vi "CalibrationFileIO.vi"(4 "Current Image Pixels":cluster{"X Pixels":i32, "Y Pixels":i32}, 6 "Calibration Type":string, 7 "CalibrationFileIO_command":enum16{"WriteSettings", "ReadSettings"}(ring), 8 "Pixel Mapping to Write":cluster{"X-PixelMap":i32[], "Y-PixelMap":i32[]}, 9 "Common Parameters IN":T1={"X.ZOOM.Compensation"=1.0, "Y.ZOOM.Compensation"=1.0, "Reso_Phase.Correction"=0.0}, 10 "Calibration paramaters_IN":T2, 11 "configuration file path":path) -> (1 "Common Parameters OUT":T1, 2 "Param Matches during a read":i32, 3 "Calibration paramaters_OUT":T2)   [LabVIEW 2012]
uses:
  Custom Controls and Typedefs/Calibration paramaters to Save.ctl
  Custom Controls and Typedefs/Calibration_commonParams.ctl
  Custom Controls and Typedefs/FGV_CalibrationKeyParams_Actions.ctl
  <vilib>/Utility/config.llb/Write Key (String).vi
  <vilib>/Utility/config.llb/Write Key (Boolean).vi
  <vilib>/Utility/config.llb/Write Key (Double).vi
  <vilib>/Utility/config.llb/Write Key (I32).vi
  <vilib>/Utility/config.llb/Read Key (Boolean).vi
  <vilib>/Utility/config.llb/Read Key (Double).vi
  <vilib>/Utility/config.llb/Read Key (I32).vi
  <vilib>/Utility/config.llb/Read Key (String).vi
  <vilib>/Utility/config.llb/NI_LVConfig.lvlib
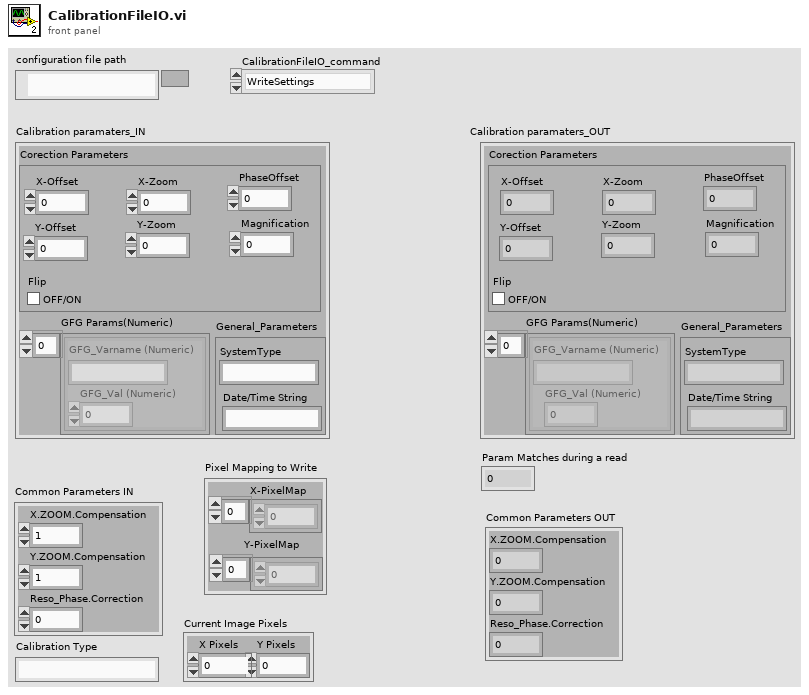
[diagram p1: front panel]
types:
  T1 = typedef "Calibration_commonParams.ctl" = cluster{"X.ZOOM.Compensation":dbl, "Y.ZOOM.Compensation":dbl, "Reso_Phase.Correction":dbl}
  T2 = typedef "Calibration paramaters to Save.ctl" = cluster{"General_Parameters":cluster{"SystemType":string, "Date/Time String":string}, "Corection Parameters":cluster{"X-Offset":i32, "Y-Offset":i32, "X-Zoom":dbl, "Y-Zoom":dbl, "PhaseOffset":dbl, "Magnification":dbl, "Flip":bool}, "GFG Params(Numeric)":cluster{"GFG_Varname (Numeric)":string, "GFG_Val (Numeric)":dbl}[]}
  T3 = typedef "FGV_CalibrationKeyParams_Actions.ctl" = enum16{"Initialize", "Grab From SciScan and Store", "Read Parameters", "ReadGFGValue"}
  T4 = typedef "NI_LVConfig.lvlib/Config Data RefNum.ctl" = refnum<k1>
  T5 = typedef "Calibration Key Param structure.ctl" = cluster{"GFG Variable Name":string, "Data Type":T6, "Value":variant}
  T6 = typedef "VariantType.lvlib/Type.ctl" = enum8{"Invalid Type", "Void", "I8", "I16", "I32", "I64", "U8", "U16", "U32", "U64", "Single Float", "Double Float", "Extended Float", "Single Complex", "Double Complex", "Extended Complex", "Enum U8", "Enum U16", "Enum U32", "Enum U64", "Single Float With Unit", "Double Float With Unit", "Extended Float With Unit", "Single Complex with Unit", "Double Complex with Unit", "Extended Complex with Unit", "Boolean", "String", "Path", "Picture", "Tag", "Array", "Cluster", "Variant", "LV Variant", "Waveform", "Timestamp", "Digital Waveform", "Digital Data", "ExpressData", "Refnum", "External Data", "VI", "Poly VI", "LabVIEW Class Instance", "Fixed Point"}
  T7 = cluster{"Key Parameters Array":T5[], "Key String":string}
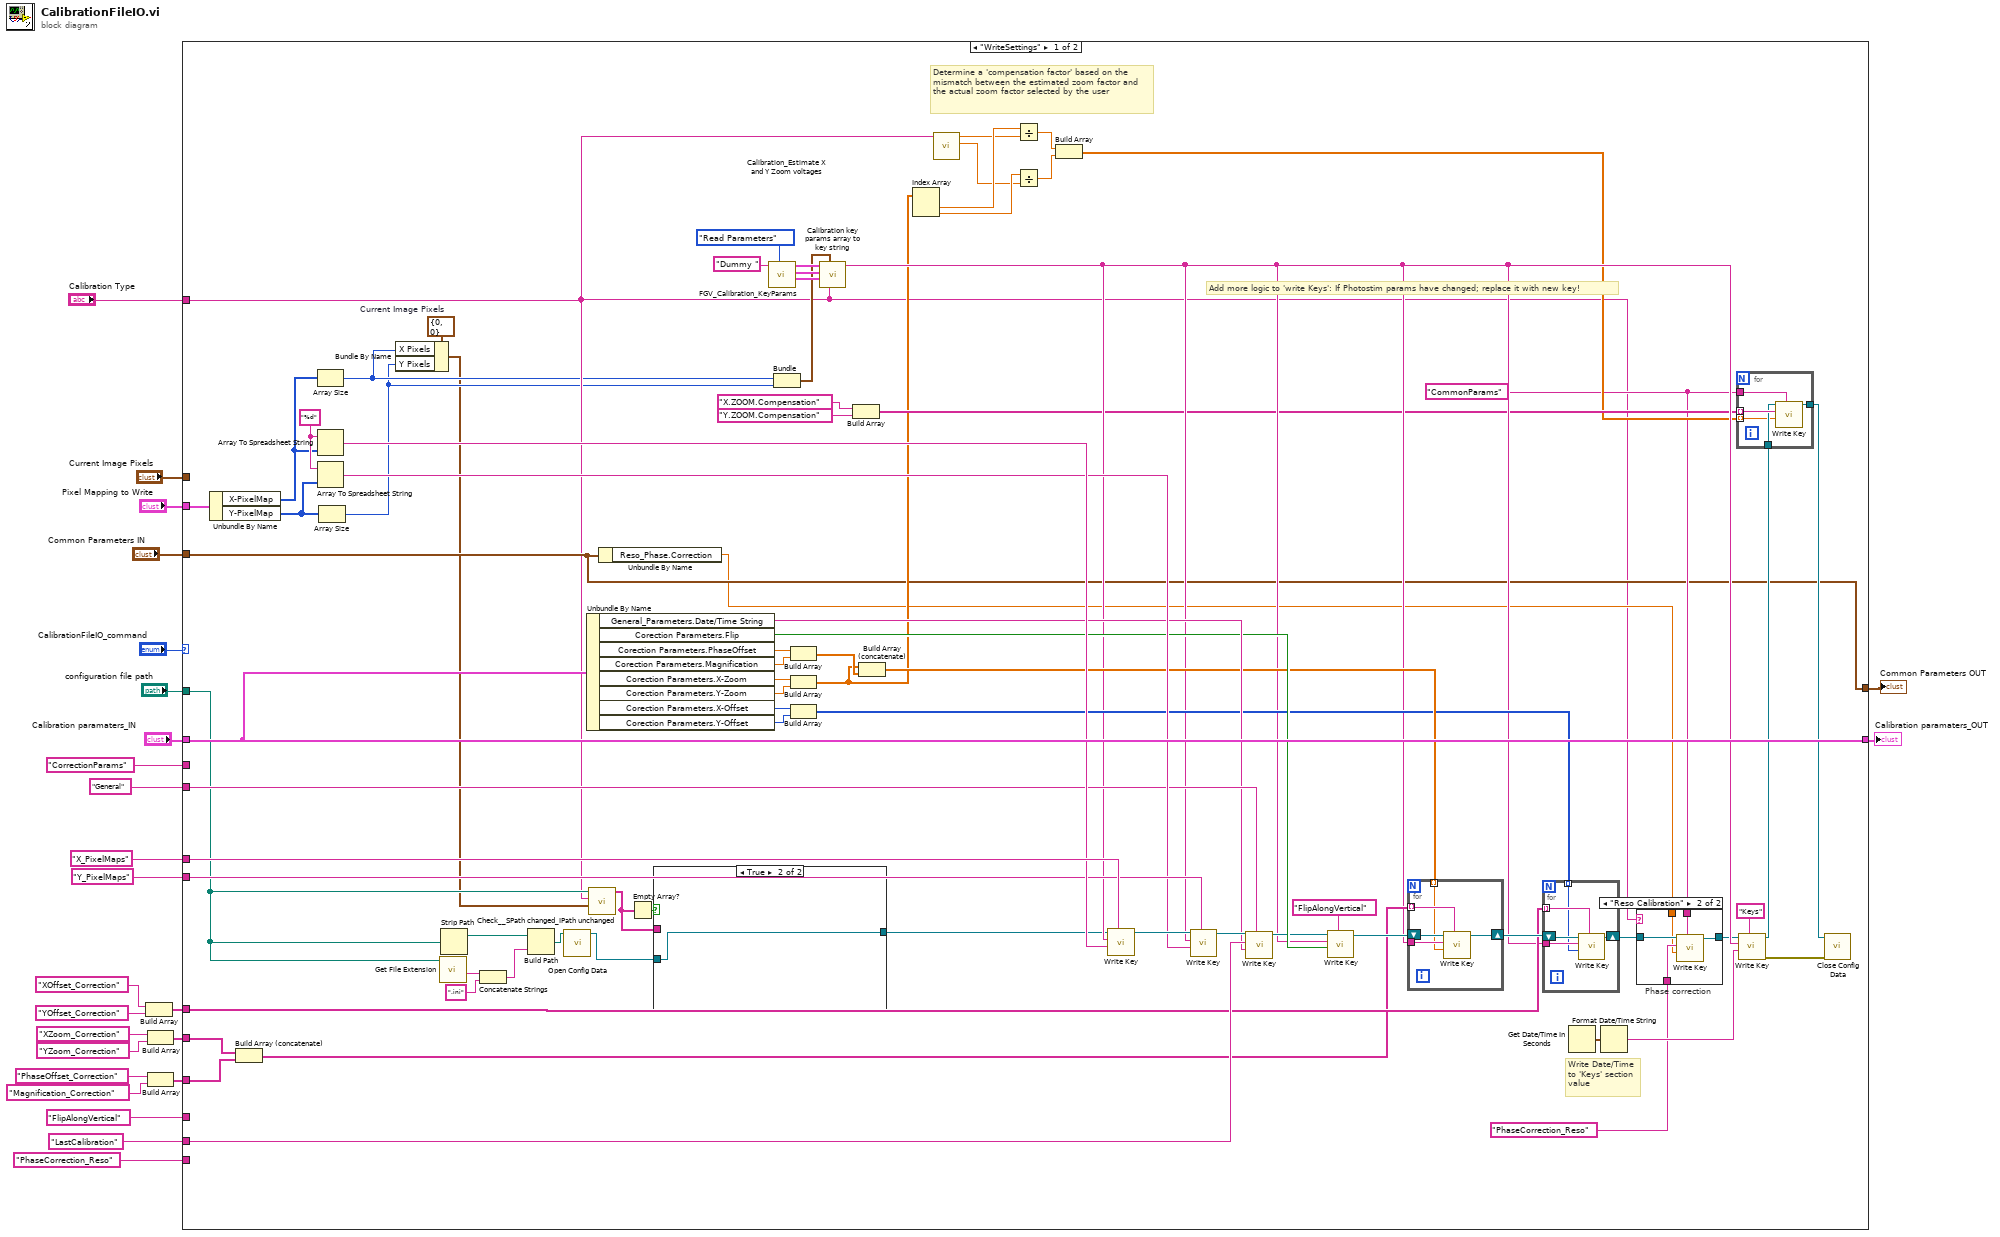
[diagram p0: block diagram]
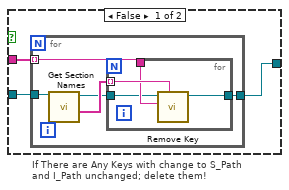
[diagram p2: hidden frame]
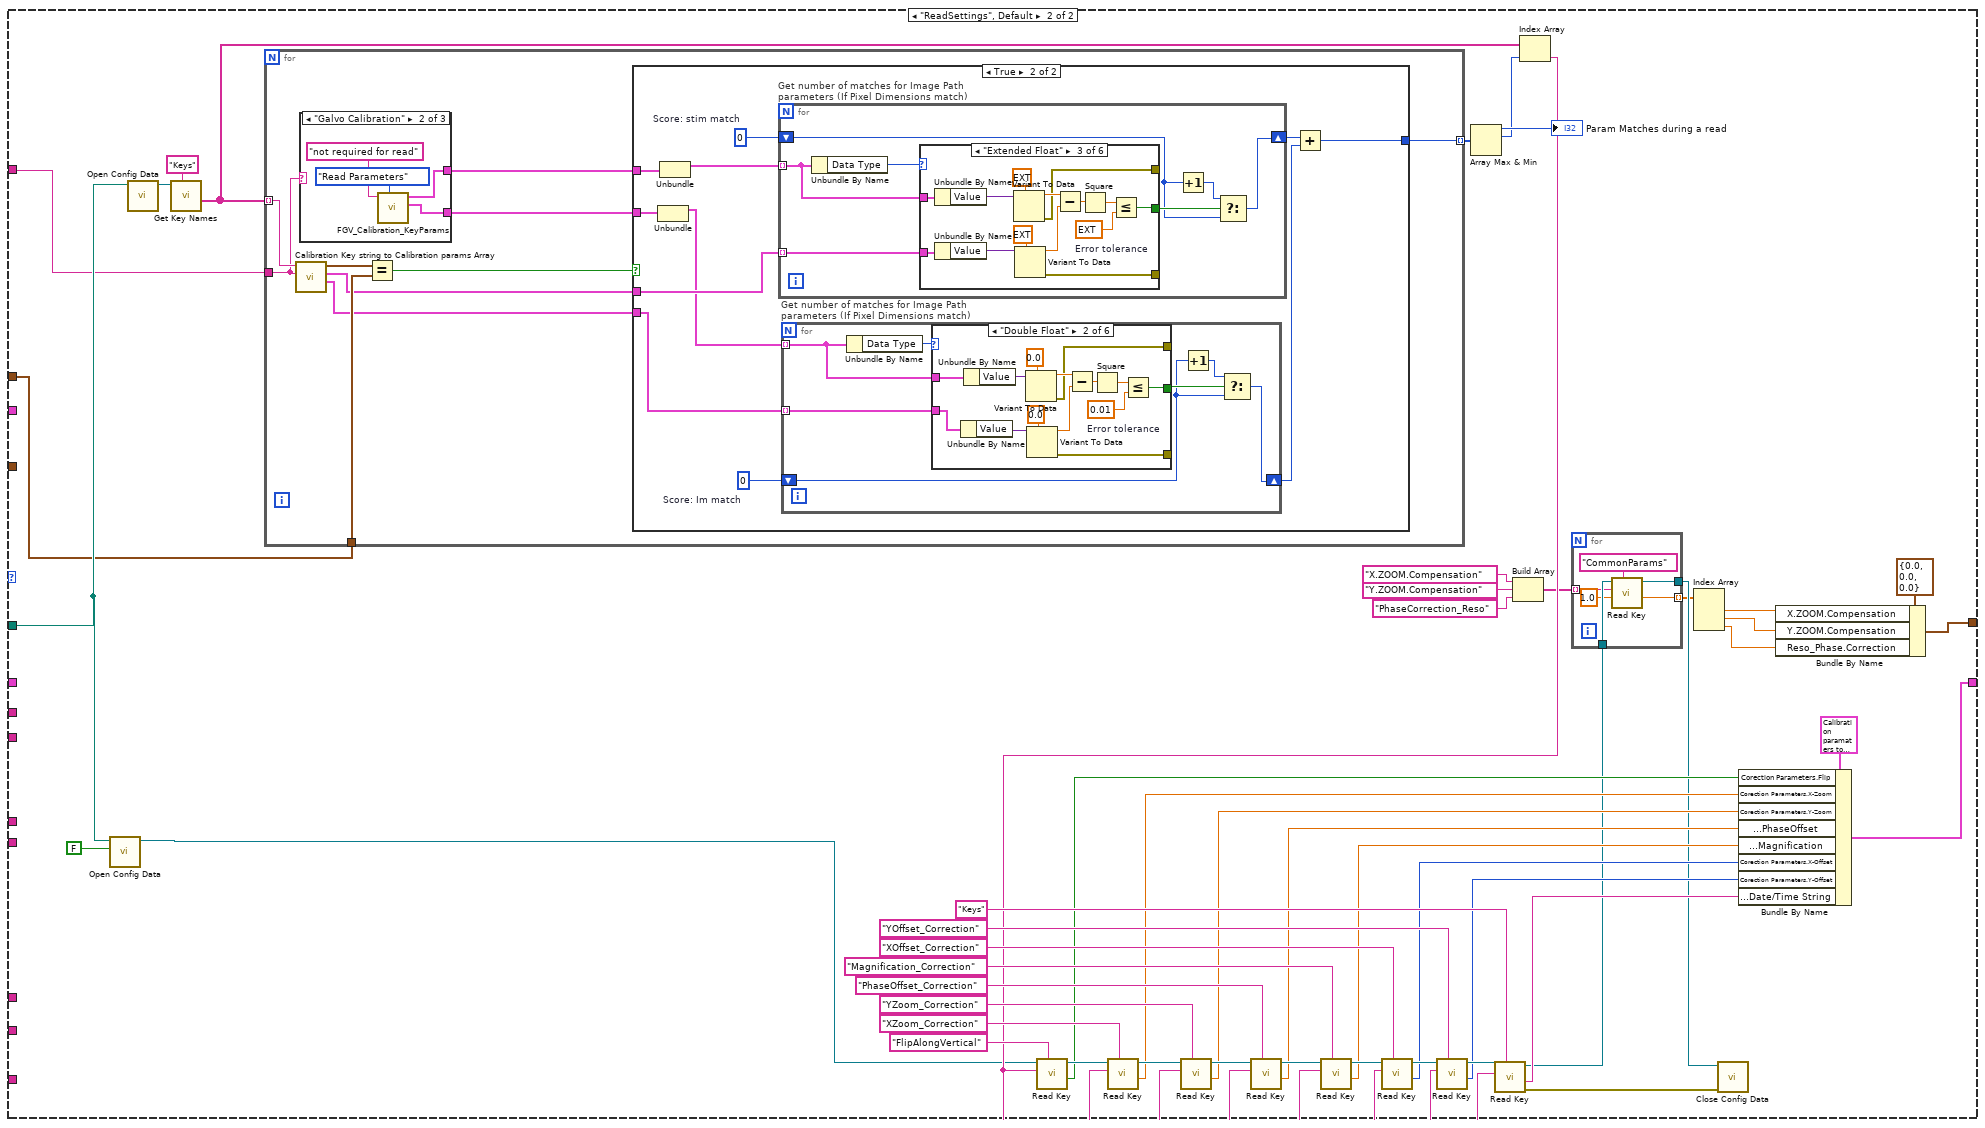
[diagram p4: hidden frame]
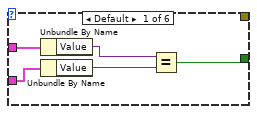
[diagram p6: hidden frame]
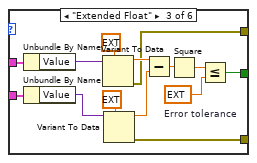
[diagram p7: hidden frame]
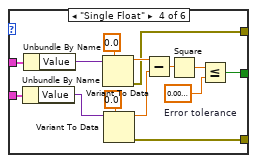
[diagram p8: hidden frame]
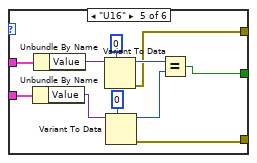
[diagram p9: hidden frame]
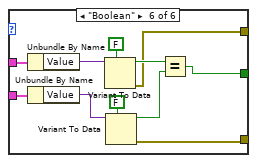
[diagram p10: hidden frame]
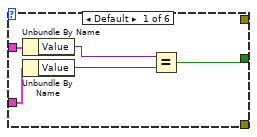
[diagram p11: hidden frame]
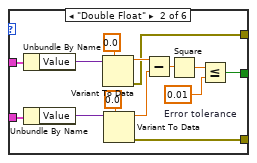
[diagram p12: hidden frame]
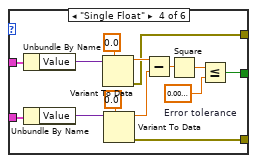
[diagram p13: hidden frame]
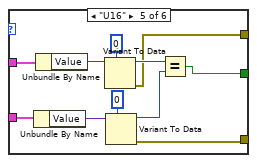
[diagram p14: hidden frame]
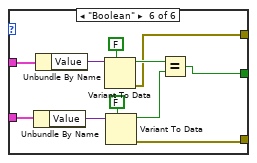
[diagram p15: hidden frame]
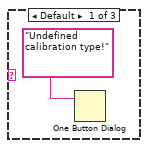
[diagram p16: hidden frame]
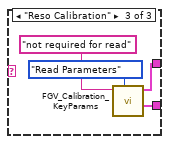
[diagram p17: hidden frame]
diagram:
  n1 = Build Array("XOffset_Correction", "YOffset_Correction") -> (w13:string[])
  n2 = Build Array("XZoom_Correction", "YZoom_Correction") -> (w14:string[])
  n3 = Build Array("PhaseOffset_Correction", "Magnification_Correction") -> (w15:string[])
  n4 = case shown="\"WriteSettings\"" "CalibrationFileIO_command" {
    tunnel: "Calibration paramaters_IN" -> [w91 _]
    tunnel: "configuration file path" -> [w35 w185]
    tunnel: "FlipAlongVertical" ("key") -> [_ _]
    tunnel: w15 -> [w67 _]
    tunnel: w14 -> [w68 _]
    tunnel: w13 -> [w63 _]
    tunnel: "CorrectionParams" -> [_ _]
    tunnel: [w91 w152] -> w11
    tunnel: "Pixel Mapping to Write" -> [w90 _]
    tunnel: "X_PixelMaps" ("section") -> [w86 _]
    tunnel: "Y_PixelMaps" ("section") -> [w83 _]
    tunnel: "General" ("section") -> [w80 _]
    tunnel: "LastCalibration" ("key") -> [w79 _]
    tunnel: "Calibration Type" -> [w34 w182]
    tunnel: "Current Image Pixels" -> [_ w181]
    tunnel: "PhaseCorrection_Reso" ("key") -> [_ _]
    tunnel: [w41 w142] -> w2
    tunnel: "Common Parameters IN" -> [w41 _]
    frame "WriteSettings" {
      w29 = cluster{"X Pixels":i32, "Y Pixels":i32} {"X Pixels"=0, "Y Pixels"=0}  # Current Image Pixels
      w42 = "CommonParams" ("section")
      w89 = "%d" ("format string")
      # "Determine a 'compensation factor' based on the mismatch between the estimated zoom factor and the actual zoom factor selected by the user"
      # "Write Date/Time to 'Keys' section value"
      # "Add more logic to 'write Keys': If Photostim params have changed; replace it with new key!"
      n5 = Unbundle By Name(w90) -> ("X-PixelMap"=w88:i32[], "Y-PixelMap"=w87:i32[])
      n6 = Build Array (concatenate)(w68, w67) -> (w56:string[])
      n7 = Array Size(array=w88) -> (size(s)=w28:i32)
      n8 = Array To Spreadsheet String(array=w88, 3:w89) -> (spreadsheet string=w85:string)  [unwired: 1 in]
      n9 = Array To Spreadsheet String(array=w87, 3:w89) -> (spreadsheet string=w82:string)  [unwired: 1 in]
      n10 = Array Size(array=w87) -> (size(s)=w27:i32)
      n11 = Bundle By Name(cluster=w29, "X Pixels"=w28, "Y Pixels"=w27) -> (w26:cluster{"X Pixels":i32, "Y Pixels":i32})
      n12 = call <vilib>:"Get File Extension.vi"("file"=w35) -> ("filename without extension"=w96:string)  [unwired: 7 in, 3 out]
      n13 = Strip Path(path=w35) -> (stripped path=w94:path)  [unwired: 1 out]
      n14 = Concatenate Strings(w96, ".ini" ("string")) -> (w93:string)
      n15 = Build Path(base path=w94, name or relative path=w93) -> (appended path=w92:path)
      n16 = call <vilib>:"Open Config Data.vi"("configuration file path"=w92) -> ("refnum"=w33:T4)  [unwired: 8 in, 2 out]
      n17 = Unbundle By Name(w91) -> ("General_Parameters.Date/Time String"=w78:string, "Corection Parameters.Flip"=w71:bool, "Corection Parameters.PhaseOffset"=w98:dbl, "Corection Parameters.Magnification"=w97:dbl, "Corection Parameters.X-Zoom"=w100:dbl, "Corection Parameters.Y-Zoom"=w99:dbl, "Corection Parameters.X-Offset"=w102:i32, "Corection Parameters.Y-Offset"=w101:i32)
      n18 = call "Check__SPath changed_IPath unchanged.vi"("Current Image Pixels"=w26, "Calibration Type"=w34, "configuration file path"=w35) -> ("Keys with S_Path change (and I_Path unchanged)"=w31:string[])  [unwired: 8 in]
      n19 = Unbundle By Name(w41) -> ("Reso_Phase.Correction"=w36:dbl)
      n20 = Empty Array?(array=w31) -> (empty?=w30:bool)
      n21 = case shown="True" w30 {
        tunnel: w31 -> [w105 _]
        tunnel: w33 -> [w104 w115]
        tunnel: [w103 w115] -> w32
        frame False {
          n22 = for "If There are Any Keys with change to S_Path and I_Path unchanged; delete them!" {
            tunnel: w105 -> [w107] mode=indexing
            tunnel: w104 -> [w110]
            tunnel: [w106] -> w103
            n23 = call <vilib>:"Get Section Names.vi"("refnum"=w110) -> ("section names"=w109:string[], "refnum out"=w108:T4)  [unwired: 8 in, 1 out]
            n24 = for {
              tunnel: w109 -> [w114] mode=indexing
              tunnel: w108 -> [w112]
              tunnel: w107 -> [w113]
              tunnel: [w111] -> w106
              n25 = call <vilib>:"Remove Key.vi"("section"=w114, "key"=w113, "refnum"=w112) -> ("refnum out"=w111:T4)  [unwired: 6 in, 2 out]
            }
          }
        }
        frame True {
        }
      }
      n26 = call "FGV_Calibration_KeyParams.vi"("Action"=FGV_CalibrationKeyParams_Actions."Read Parameters", "System Type"="Dummy ") -> ("Imaging Reso Key Parameters"=w73:T7, "Imaging Galvo Key Parameters"=w74:T7, "Stimulating Galvo Key Parameters"=w75:T7)  [unwired: 4 in, 3 out]
      n27 = Bundle(w28, w27) -> (w62:cluster{i32, i32})  [unwired: 1 in]
      n28 = Build Array(w98, w97) -> (w57:dbl[])
      n29 = Build Array(w100, w99) -> (w47:dbl[])
      n30 = Build Array(w102, w101) -> (w64:i32[])
      n31 = call "Calibration key params array to key string.vi"("Calibration Type"=w34, "Pixels"=w62, "Imaging Reso Key Parameters"=w73, "Imaging Galvo Key Parameters"=w74, "Stimulating Galvo Key Parameters"=w75) -> ("Key String Out"=w55:string)  [unwired: 6 in]
      n32 = Build Array("X.ZOOM.Compensation" ("section"), "Y.ZOOM.Compensation" ("section")) -> (w50:string[])
      n33 = Build Array (concatenate)(w47, w57) -> (w66:dbl[])
      n34 = Index Array(array=w47) -> (element #1=w46:dbl, element #2=w45:dbl)  [unwired: 2 in]
      n35 = call "Calibration_Estimate X and Y Zoom voltages.vi"("System Type"=w34) -> ("Y.ZOOM_estimated"=w37:dbl, "X.ZOOM_estimated"=w38:dbl)  [unwired: 9 in]
      n36 = Divide(x=w46, y=w38) -> (x/y=w39:dbl)
      n37 = Divide(x=w45, y=w37) -> (x/y=w40:dbl)
      n38 = Build Array(w39, w40) -> (w44:dbl[])
      n39 = call-poly <vilib>:"Write Key.vi"("section"=w86, "value"=w85, "key"=w55, "refnum"=w32) -> ("refnum out"=w84:T4)  [unwired: 5 in, 2 out]
      n40 = call-poly <vilib>:"Write Key.vi"("section"=w83, "value"=w82, "key"=w55, "refnum"=w84) -> ("refnum out"=w81:T4)  [unwired: 5 in, 2 out]
      n41 = call-poly <vilib>:"Write Key.vi"("section"=w80, "value"=w78, "key"=w79, "refnum"=w81) -> ("refnum out"=w69:T4)  [unwired: 5 in, 2 out]
      n42 = call-poly <vilib>:"Write Key.vi"("section"="FlipAlongVertical", "value"=w71, "key"=w55, "refnum"=w69) -> ("refnum out"=w70:T4)  [unwired: 5 in, 2 out]
      n43 = for {
        tunnel: w55 -> [w136]
        tunnel: w56 -> [w133] mode=indexing
        shift-right: [w134] -> w65
        shift-left: w70 -> [w135]
        tunnel: w66 -> [w132] mode=indexing
        n44 = call-poly <vilib>:"Write Key.vi"("section"=w133, "value"=w132, "key"=w136, "refnum"=w135) -> ("refnum out"=w134:T4)  [unwired: 5 in, 2 out]
      }
      n45 = for {
        tunnel: w55 -> [w131]
        tunnel: w63 -> [w128] mode=indexing
        shift-right: [w129] -> w54
        shift-left: w65 -> [w130]
        tunnel: w64 -> [w127] mode=indexing
        n46 = call-poly <vilib>:"Write Key.vi"("section"=w128, "value"=w127, "key"=w131, "refnum"=w130) -> ("refnum out"=w129:T4)  [unwired: 5 in, 2 out]
      }
      n47 = Get Date/Time In Seconds() -> (seconds since 1Jan1904=w59:timestamp)
      n48 = Format Date/Time String(seconds (now)=w59) -> (date/time string=w58:string)  [unwired: 2 in]
      n49 = case "Phase correction" shown="\"Reso Calibration\"" w34 {
        tunnel: "PhaseCorrection_Reso" ("section") -> [_ w124]
        tunnel: w54 -> [w121 w125]
        tunnel: [w121 w126] -> w53
        tunnel: w42 -> [_ w123]
        tunnel: w36 -> [_ w122]
        frame "False", Default {
        }
        frame "Reso Calibration" {
          n50 = call-poly <vilib>:"Write Key.vi"("section"=w123, "value"=w122, "key"=w124, "refnum"=w125) -> ("refnum out"=w126:T4)  [unwired: 5 in, 2 out]
        }
      }
      n51 = call-poly <vilib>:"Write Key.vi"("section"="Keys", "value"=w58, "key"=w55, "refnum"=w53) -> ("error out"=w60:errorcluster, "refnum out"=w49:T4)  [unwired: 5 in, 1 out]
      n52 = for {
        tunnel: w49 -> [w118]
        tunnel: w50 -> [w120] mode=indexing
        tunnel: [w119] -> w48
        tunnel: w44 -> [w117] mode=indexing
        tunnel: w42 -> [w116]
        n53 = call-poly <vilib>:"Write Key.vi"("section"=w116, "value"=w117, "key"=w120, "refnum"=w118) -> ("refnum out"=w119:T4)  [unwired: 5 in, 2 out]
      }
      n54 = call <vilib>:"Close Config Data.vi"("error in (no error)"=w60, "refnum"=w48) -> ()  [unwired: 8 in, 2 out]
    }
    frame "ReadSettings", Default {
      n55 = call <vilib>:"Open Config Data.vi"("create file if necessary (T)"=FALSE, "configuration file path"=w185) -> ("refnum"=w141:T4)  [unwired: 7 in, 2 out]
      n56 = call <vilib>:"Open Config Data.vi"("configuration file path"=w185) -> ("refnum"=w183:T4)  [unwired: 8 in, 2 out]
      n57 = call <vilib>:"Get Key Names.vi"("section"="Keys", "refnum"=w183) -> ("key names"=w179:string[])  [unwired: 6 in, 3 out]
      n58 = for {
        tunnel: w179 -> [w202] mode=indexing
        tunnel: w182 -> [w201]
        tunnel: w181 -> [w199]
        tunnel: [w193] -> w177 mode=indexing
        n59 = call "Calibration Key string to Calibration params Array.vi"("Calibration Type"=w201, "Key String IN"=w202) -> ("Imaging (Galvo/Reso) Key Array"=w196:T5[], "Photostim Galvo Key Array"=w197:T5[], "Image Pixels OUT"=w200:cluster{"X Pixels":i32, "Y Pixels":i32})  [unwired: 7 in]
        n60 = case shown="\"Galvo Calibration\"" w201 {
          tunnel: [_ w368 w372] -> w195
          tunnel: [_ w367 w371] -> w194
          frame Default {
            n61 = One Button Dialog(message="Undefined calibration type!") -> ()  [unwired: 1 in, 1 out]
          }
          frame "Galvo Calibration" {
            n62 = call "FGV_Calibration_KeyParams.vi"("Action"=FGV_CalibrationKeyParams_Actions."Read Parameters", "System Type"="not required for read") -> ("Imaging Galvo Key Parameters"=w367:T7, "Stimulating Galvo Key Parameters"=w368:T7)  [unwired: 4 in, 4 out]
          }
          frame "Reso Calibration" {
            n63 = call "FGV_Calibration_KeyParams.vi"("Action"=FGV_CalibrationKeyParams_Actions."Read Parameters", "System Type"="not required for read") -> ("Imaging Reso Key Parameters"=w371:T7, "Stimulating Galvo Key Parameters"=w372:T7)  [unwired: 4 in, 4 out]
          }
        }
        n64 = Equal?(x=w200, y=w199) -> (x = y?=w198:bool)
        n65 = case shown="True" w198 {
          tunnel: w197 -> [_ w210]
          tunnel: w196 -> [_ w205]
          tunnel: w195 -> [_ w213]
          tunnel: w194 -> [_ w212]
          tunnel: [_ w207] -> w193
          frame False {
          }
          frame True {
            w204 = 0  # Score: Im match
            w209 = 0  # Score: stim match
            n66 = Unbundle(w212) -> ("Key Parameters Array"=w206:T5[])  [unwired: 1 out]
            n67 = Unbundle(w213) -> ("Key Parameters Array"=w211:T5[])  [unwired: 1 out]
            n68 = for "Get number of matches for Image Path parameters (If Pixel Dimensions match)" {
              tunnel: w211 -> [w295] mode=indexing
              tunnel: w210 -> [w294] mode=indexing
              shift-right: [w290] -> w208
              shift-left: w209 -> [w291]
              n69 = Unbundle By Name(w295) -> ("Data Type"=w296:T6)
              n70 = case shown="\"Extended Float\"" w296 {
                tunnel: w294 -> [w301 w314 w328 w342 w353 w364]
                tunnel: [w298 w304 w318 w332 w346 w359] -> w293
                tunnel: w295 -> [w297 w315 w329 w343 w354 w365]
                tunnel: [_ w303 w316 w331 w345 w356] -> _
                tunnel: [_ w302 w317 w330 w344 w355] -> _
                frame Default {
                  n71 = Unbundle By Name(w297) -> ("Value"=w300:variant)
                  n72 = Unbundle By Name(w301) -> ("Value"=w299:variant)
                  n73 = Equal?(x=w300, y=w299) -> (x = y?=w298:bool)
                }
                frame "Double Float" {
                  w306 = 0.01  # Error tolerance
                  n74 = Unbundle By Name(w315) -> ("Value"=w313:variant)
                  n75 = Unbundle By Name(w314) -> ("Value"=w310:variant)
                  n76 = Variant To Data(type=0.0, Variant=w313) -> (data=w309:dbl, error out=w303:errorcluster)  [unwired: 1 in]
                  n77 = Variant To Data(type=0.0, Variant=w310) -> (data=w308:dbl, error out=w302:errorcluster)  [unwired: 1 in]
                  n78 = Subtract(x=w309, y=w308) -> (x-y=w307:dbl)
                  n79 = Square(x=w307) -> (x^2=w305:dbl)
                  n80 = Less Or Equal?(x=w305, y=w306) -> (x <= y?=w304:bool)
                }
                frame "Extended Float" {
                  w320 = ext 0.01  # Error tolerance
                  n81 = Unbundle By Name(w329) -> ("Value"=w327:variant)
                  n82 = Unbundle By Name(w328) -> ("Value"=w324:variant)
                  n83 = Variant To Data(type=ext 0.0, Variant=w327) -> (data=w323:ext, error out=w316:errorcluster)  [unwired: 1 in]
                  n84 = Variant To Data(type=ext 0.0, Variant=w324) -> (data=w322:ext, error out=w317:errorcluster)  [unwired: 1 in]
                  n85 = Subtract(x=w323, y=w322) -> (x-y=w321:ext)
                  n86 = Square(x=w321) -> (x^2=w319:ext)
                  n87 = Less Or Equal?(x=w319, y=w320) -> (x <= y?=w318:bool)
                }
                frame "Single Float" {
                  w334 = sgl 0.01  # Error tolerance
                  n88 = Unbundle By Name(w343) -> ("Value"=w341:variant)
                  n89 = Unbundle By Name(w342) -> ("Value"=w338:variant)
                  n90 = Variant To Data(type=sgl 0.0, Variant=w341) -> (data=w337:sgl, error out=w331:errorcluster)  [unwired: 1 in]
                  n91 = Variant To Data(type=sgl 0.0, Variant=w338) -> (data=w336:sgl, error out=w330:errorcluster)  [unwired: 1 in]
                  n92 = Subtract(x=w337, y=w336) -> (x-y=w335:sgl)
                  n93 = Square(x=w335) -> (x^2=w333:sgl)
                  n94 = Less Or Equal?(x=w333, y=w334) -> (x <= y?=w332:bool)
                }
                frame "U16" {
                  n95 = Unbundle By Name(w353) -> ("Value"=w349:variant)
                  n96 = Unbundle By Name(w354) -> ("Value"=w351:variant)
                  n97 = Variant To Data(type=u16 0, Variant=w351) -> (data=w348:u16, error out=w345:errorcluster)  [unwired: 1 in]
                  n98 = Variant To Data(type=u16 0, Variant=w349) -> (data=w347:u16, error out=w344:errorcluster)  [unwired: 1 in]
                  n99 = Equal?(x=w348, y=w347) -> (x = y?=w346:bool)
                }
                frame "Boolean" {
                  n100 = Unbundle By Name(w364) -> ("Value"=w362:variant)
                  n101 = Unbundle By Name(w365) -> ("Value"=w363:variant)
                  n102 = Variant To Data(type=FALSE, Variant=w363) -> (data=w361:bool, error out=w356:errorcluster)  [unwired: 1 in]
                  n103 = Variant To Data(type=FALSE, Variant=w362) -> (data=w360:bool, error out=w355:errorcluster)  [unwired: 1 in]
                  n104 = Equal?(x=w361, y=w360) -> (x = y?=w359:bool)
                }
              }
              n105 = Increment(x=w291) -> (x+1=w292:i32)
              n106 = Select(t=w292, s=w293, f=w291) -> (s? t:f=w290:i32)
            }
            n107 = for "Get number of matches for Image Path parameters (If Pixel Dimensions match)" {
              shift-right: [w217] -> w203
              shift-left: w204 -> [w216]
              tunnel: w206 -> [w215] mode=indexing
              tunnel: w205 -> [w214] mode=indexing
              n108 = Unbundle By Name(w215) -> ("Data Type"=w218:T6)
              n109 = case shown="\"Double Float\"" w218 {
                tunnel: [w223 w229 w243 w257 w271 w284] -> w220
                tunnel: w215 -> [w222 w239 w253 w267 w278 w289]
                tunnel: w214 -> [w221 w228 w242 w256 w270 w281]
                tunnel: [_ w227 w240 w255 w269 w280] -> _
                tunnel: [_ w226 w241 w254 w268 w279] -> _
                frame Default {
                  n110 = Unbundle By Name(w222) -> ("Value"=w225:variant)
                  n111 = Unbundle By Name(w221) -> ("Value"=w224:variant)
                  n112 = Equal?(x=w225, y=w224) -> (x = y?=w223:bool)
                }
                frame "Double Float" {
                  w231 = 0.01  # Error tolerance
                  n113 = Unbundle By Name(w228) -> ("Value"=w235:variant)
                  n114 = Unbundle By Name(w239) -> ("Value"=w238:variant)
                  n115 = Variant To Data(type=0.0, Variant=w238) -> (data=w234:dbl, error out=w227:errorcluster)  [unwired: 1 in]
                  n116 = Variant To Data(type=0.0, Variant=w235) -> (data=w233:dbl, error out=w226:errorcluster)  [unwired: 1 in]
                  n117 = Subtract(x=w234, y=w233) -> (x-y=w232:dbl)
                  n118 = Square(x=w232) -> (x^2=w230:dbl)
                  n119 = Less Or Equal?(x=w230, y=w231) -> (x <= y?=w229:bool)
                }
                frame "Extended Float" {
                  w245 = ext 0.01  # Error tolerance
                  n120 = Unbundle By Name(w253) -> ("Value"=w252:variant)
                  n121 = Unbundle By Name(w242) -> ("Value"=w249:variant)
                  n122 = Variant To Data(type=ext 0.0, Variant=w252) -> (data=w248:ext, error out=w240:errorcluster)  [unwired: 1 in]
                  n123 = Variant To Data(type=ext 0.0, Variant=w249) -> (data=w247:ext, error out=w241:errorcluster)  [unwired: 1 in]
                  n124 = Subtract(x=w248, y=w247) -> (x-y=w246:ext)
                  n125 = Square(x=w246) -> (x^2=w244:ext)
                  n126 = Less Or Equal?(x=w244, y=w245) -> (x <= y?=w243:bool)
                }
                frame "Single Float" {
                  w259 = sgl 0.01  # Error tolerance
                  n127 = Unbundle By Name(w256) -> ("Value"=w263:variant)
                  n128 = Unbundle By Name(w267) -> ("Value"=w266:variant)
                  n129 = Variant To Data(type=sgl 0.0, Variant=w266) -> (data=w262:sgl, error out=w255:errorcluster)  [unwired: 1 in]
                  n130 = Variant To Data(type=sgl 0.0, Variant=w263) -> (data=w261:sgl, error out=w254:errorcluster)  [unwired: 1 in]
                  n131 = Subtract(x=w262, y=w261) -> (x-y=w260:sgl)
                  n132 = Square(x=w260) -> (x^2=w258:sgl)
                  n133 = Less Or Equal?(x=w258, y=w259) -> (x <= y?=w257:bool)
                }
                frame "U16" {
                  n134 = Unbundle By Name(w270) -> ("Value"=w274:variant)
                  n135 = Unbundle By Name(w278) -> ("Value"=w276:variant)
                  n136 = Variant To Data(type=u16 0, Variant=w276) -> (data=w273:u16, error out=w269:errorcluster)  [unwired: 1 in]
                  n137 = Variant To Data(type=u16 0, Variant=w274) -> (data=w272:u16, error out=w268:errorcluster)  [unwired: 1 in]
                  n138 = Equal?(x=w273, y=w272) -> (x = y?=w271:bool)
                }
                frame "Boolean" {
                  n139 = Unbundle By Name(w289) -> ("Value"=w288:variant)
                  n140 = Unbundle By Name(w281) -> ("Value"=w287:variant)
                  n141 = Variant To Data(type=FALSE, Variant=w288) -> (data=w286:bool, error out=w280:errorcluster)  [unwired: 1 in]
                  n142 = Variant To Data(type=FALSE, Variant=w287) -> (data=w285:bool, error out=w279:errorcluster)  [unwired: 1 in]
                  n143 = Equal?(x=w286, y=w285) -> (x = y?=w284:bool)
                }
              }
              n144 = Increment(x=w216) -> (x+1=w219:i32)
              n145 = Select(t=w219, s=w220, f=w216) -> (s? t:f=w217:i32)
            }
            n146 = Add(x=w208, y=w203) -> (x+y=w207:i32)
          }
        }
      }
      n147 = Array Max & Min(array=w177) -> (max value=→"Param Matches during a read":i32, max index (indices)=w178:i32)  [unwired: 2 out]
      n148 = Build Array("X.ZOOM.Compensation" ("section"), "Y.ZOOM.Compensation" ("section"), "PhaseCorrection_Reso" ("section")) -> (w147:string[])
      n149 = Index Array(array=w179, index=w178) -> (element=w151:string)
      n150 = call-poly <vilib>:"Read Key.vi"("section"="FlipAlongVertical", "key"=w151, "refnum"=w141) -> ("value"=w153:bool, "refnum out"=w171:T4)  [unwired: 5 in, 2 out]
      n151 = call-poly <vilib>:"Read Key.vi"("section"="XZoom_Correction", "key"=w151, "refnum"=w171) -> ("value"=w154:dbl, "refnum out"=w170:T4)  [unwired: 5 in, 2 out]
      n152 = call-poly <vilib>:"Read Key.vi"("section"="YZoom_Correction", "key"=w151, "refnum"=w170) -> ("value"=w155:dbl, "refnum out"=w169:T4)  [unwired: 5 in, 2 out]
      n153 = call-poly <vilib>:"Read Key.vi"("section"="PhaseOffset_Correction", "key"=w151, "refnum"=w169) -> ("value"=w156:dbl, "refnum out"=w168:T4)  [unwired: 5 in, 2 out]
      n154 = call-poly <vilib>:"Read Key.vi"("section"="Magnification_Correction", "key"=w151, "refnum"=w168) -> ("value"=w157:dbl, "refnum out"=w167:T4)  [unwired: 5 in, 2 out]
      n155 = call-poly <vilib>:"Read Key.vi"("section"="XOffset_Correction", "key"=w151, "refnum"=w167) -> ("value"=w158:i32, "refnum out"=w166:T4)  [unwired: 5 in, 2 out]
      n156 = call-poly <vilib>:"Read Key.vi"("section"="YOffset_Correction", "key"=w151, "refnum"=w166) -> ("value"=w159:i32, "refnum out"=w161:T4)  [unwired: 5 in, 2 out]
      n157 = call-poly <vilib>:"Read Key.vi"("section"="Keys", "key"=w151, "refnum"=w161) -> ("error out"=w138:errorcluster, "value"=w160:string, "refnum out"=w137:T4)  [unwired: 5 in, 1 out]
      n158 = for {
        tunnel: w137 -> [w191]
        tunnel: w147 -> [w190] mode=indexing
        tunnel: [w189] -> w146
        tunnel: [w188] -> w145 mode=indexing
        n159 = call-poly <vilib>:"Read Key.vi"("section"="CommonParams", "default value"=1.0, "key"=w190, "refnum"=w191) -> ("value"=w188:dbl, "refnum out"=w189:T4)  [unwired: 4 in, 2 out]
      }
      n160 = Index Array(array=w145) -> (element #1=w144:dbl, element #2=w143:dbl, element #3=w139:dbl)  [unwired: 3 in]
      n161 = call <vilib>:"Close Config Data.vi"("error in (no error)"=w138, "refnum"=w146) -> ()  [unwired: 8 in, 2 out]
      n162 = Bundle By Name(cluster=T2 {"General_Parameters"={"SystemType"="", "Date/Time String"=""}, "Corection Parameters"={"X-Offset"=0, "Y-Offset"=0, "X-Zoom"=0.0, "Y-Zoom"=0.0, "PhaseOffset"=0.0, "Magnification"=0.0, "Flip"=FALSE}, "GFG Params(Numeric)"=[]} ("Calibration paramaters_OUT"), "Corection Parameters.Flip"=w153, "Corection Parameters.X-Zoom"=w154, "Corection Parameters.Y-Zoom"=w155, "Corection Parameters.PhaseOffset"=w156, "Corection Parameters.Magnification"=w157, "Corection Parameters.X-Offset"=w158, "Corection Parameters.Y-Offset"=w159, "General_Parameters.Date/Time String"=w160) -> (w152:T2)
      n163 = Bundle By Name(cluster=T1 {"X.ZOOM.Compensation"=0.0, "Y.ZOOM.Compensation"=0.0, "Reso_Phase.Correction"=0.0} ("Common Parameters IN"), "X.ZOOM.Compensation"=w144, "Y.ZOOM.Compensation"=w143, "Reso_Phase.Correction"=w139) -> (w142:T1)
    }
  }
  "Calibration paramaters_OUT" <- w11
  "Common Parameters OUT" <- w2
